vi "TCP Write.vi"(8 "error in (no error)":errorcluster, 9 "timeout ms (25000)":i32=25000, 10 "Write Data":string, 11 "connection ID In":refnum<k5>) -> (0 "error out":errorcluster, 3 "connection ID Out":refnum<k5>)   [LabVIEW 2014, in "SLL Easy API via TCP.lvclass"]
doc: "Executes a TCP Write Operation, prefixing the size of the data being transmitted at the beginning."
uses:
  SLL Easy API via TCP.lvclass
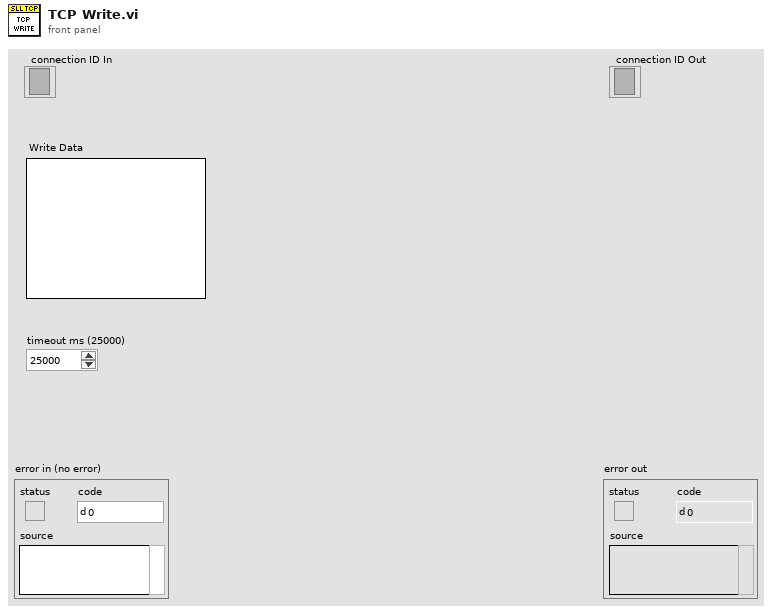
[diagram p1: front panel]
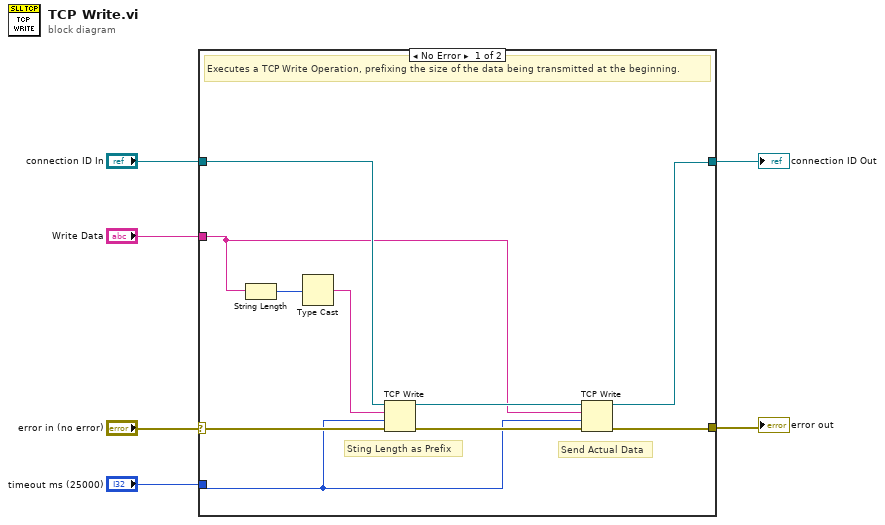
[diagram p0: block diagram]
diagram:
  n1 = case shown="No Error" "error in (no error)" {
    selector: "error in (no error)" -> [w16 w18]
    tunnel: "connection ID In" -> [w15 w17]
    tunnel: [w10 w18] -> w4
    tunnel: "Write Data" -> [w7 _]
    tunnel: [w9 w17] -> w2
    tunnel: "timeout ms (25000)" -> [w8 _]
    frame No Error {
      # "Send Actual Data"
      # "Sting Length as Prefix"
      # "Executes a TCP Write Operation, prefixing the size of the data being transmitted at the beginning."
      n2 = String Length(string=w7) -> (length=w14:i32)
      n3 = Type Cast(x=w14) -> (*(type *) &x=w13:string)  [unwired: 1 in]
      n4 = TCP Write(connection ID=w15, data in=w13, error in (no error)=w16, 9:w8) -> (connection ID out=w11:refnum<k5>, error out=w12:errorcluster)  [unwired: 1 out]
      n5 = TCP Write(connection ID=w11, data in=w7, error in (no error)=w12, 9:w8) -> (connection ID out=w9:refnum<k5>, error out=w10:errorcluster)  [unwired: 1 out]
    }
    frame Error {
    }
  }
  "error out" <- w4
  "connection ID Out" <- w2
